vi "Script Unflatten VI.vi"(4 "Message Paths":T5, 6 "Message":T1, 7 "App":refnum<vi>, 8 "error in (no error)":errorcluster, 11 "LV-Protoc in":refnum<class "LV-Protoc.lvclass">) -> (0 "error out":errorcluster, 3 "LV-Protoc out":refnum<class "LV-Protoc.lvclass">)   [LabVIEW 2020, in "LV-Protoc.lvlib" / "LV-Protoc.lvclass"]
uses:
  LV-Protoc.lvclass
  Message Paths.ctl
  LV-Proto/Message.ctl
  LV-Proto/Field.ctl
  LV-Proto/Type.ctl
  LV-Proto/Proto Type.ctl
  LV-Protoc.lvlib
  LV-Proto/LV-Proto.lvlib
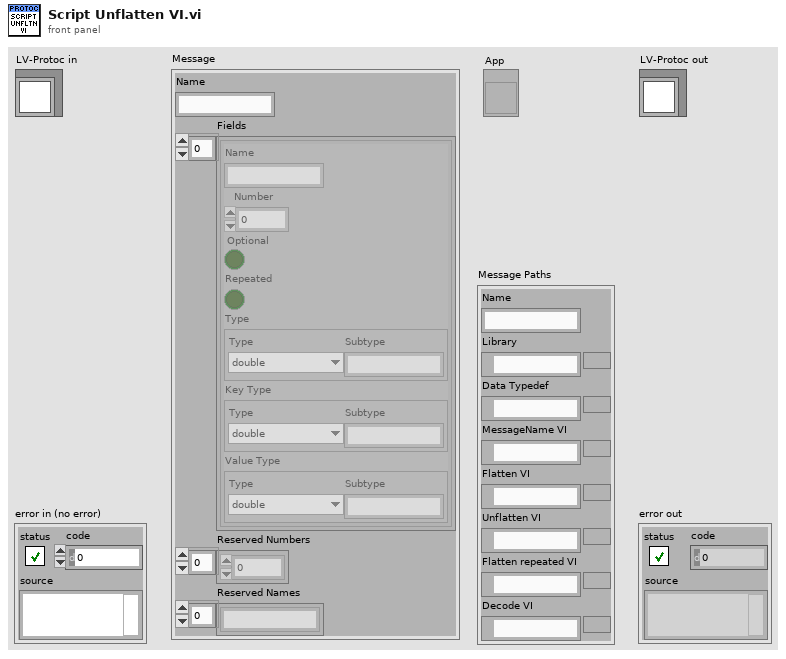
[diagram p1: front panel]
types:
  T1 = typedef "LV-Proto.lvlib/Message.ctl" = cluster{"Name":string, "Fields":T2[], "Reserved Numbers":u32[], "Reserved Names":string[]}
  T2 = typedef "LV-Proto.lvlib/Field.ctl" = cluster{"Name":string, "Number":u32, "Optional":bool, "Repeated":bool, "Type":T3, "Key Type":T3, "Value Type":T3}
  T3 = typedef "LV-Proto.lvlib/Type.ctl" = cluster{"Type":T4, "Subtype":string}
  T4 = typedef "LV-Proto.lvlib/Proto Type.ctl" = enum16{"UNKNOWN", "double", "float", "int32", "int64", "uint32", "uint64", "sint32", "sint64", "fixed32", "fixed64", "sfixed32", "sfixed64", "bool", "string", "bytes", "enum", "map", "message"}
  T5 = typedef "LV-Protoc.lvlib/Message Paths.ctl" = cluster{"Name":string, "Library":path, "Data Typedef":path, "MessageName VI":path, "Flatten VI":path, "Unflatten VI":path, "Flatten repeated VI":path, "Decode VI":path}
  T6 = typedef "LV-Protoc.lvlib/Unflatten Refs.ctl" = cluster{"VI":refnum<vi>, "BD":refnum<vi>, "Case":refnum<vi>, "Selector":refnum<vi>, "Data":refnum<vi>, "Type":refnum<vi>}
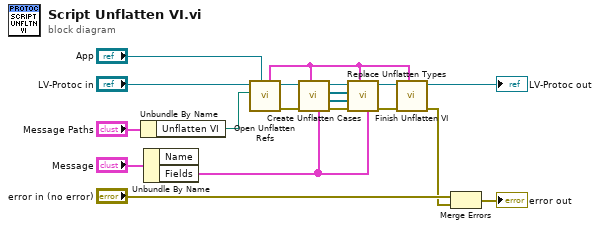
[diagram p0: block diagram]
diagram:
  n1 = Unbundle By Name("Message Paths") -> ("Unflatten VI"=w13:path)
  n2 = Unbundle By Name("Message") -> ("Fields"=w6:T2[])  [unwired: 1 out]
  n3 = call "Open Unflatten Refs.vi"("App"="App", "VI Path"=w13, "LV-Protoc in"="LV-Protoc in") -> ("error out"=w11:errorcluster, "LV-Protoc out"=w14:refnum<class "LV-Protoc.lvclass">, "Unflatten Refs"=w3:T6)  [unwired: 6 in]
  n4 = call "Create Unflatten Cases.vi"("Fields"=w6, "Unflatten Refs"=w3, "error in (no error)"=w11, "LV-Protoc in"=w14) -> ("error out"=w9:errorcluster, "Bundlers"=w7:refnum<vi>[], "Decodes"=w8:refnum<vi>[], "LV-Protoc out"=w12:refnum<class "LV-Protoc.lvclass">)  [unwired: 4 in]
  n5 = call "Replace Unflatten Types.vi"("Fields"=w6, "Unflatten Refs"=w3, "error in (no error)"=w9, "Bundlers"=w7, "Decodes"=w8, "LV-Protoc in"=w12) -> ("error out"=w4:errorcluster, "LV-Protoc out"=w10:refnum<class "LV-Protoc.lvclass">)  [unwired: 4 in]
  n6 = call "Finish Unflatten VI.vi"("Unflatten Refs"=w3, "error in (no error)"=w4, "LV-Protoc in"=w10) -> ("error out"=w2:errorcluster, "LV-Protoc out"=→"LV-Protoc out":refnum<class "LV-Protoc.lvclass">)  [unwired: 7 in]
  n7 = Merge Errors("error in (no error)", w2) -> (→"error out":errorcluster)
